vi "Get Waveform Name and Units.vi"(8 "Error In":errorcluster, 10 "CD Settings":T2={"CD Task Dependency"=18446744073709551615, "CD Task Dependency Ref"=18446744073709551615, "CD Task Available Wfms"=[], "CD Task Selected Wfms"=[], "Buffer Length (samples)"=0, "Min Enabled"=FALSE, "Max Enabled "=FALSE, "SP Enabled"=FALSE, "RMS Enabled"=FALSE, "Buffer Length (s)"=0.0, "Task Rate"=0.0, "Number of DAQ Chanels"=0} {"CD Task Dependency Ref" format="%.0x"; "CD Task Dependency" format="%.0x"}, 11 "CustomDevice Ref":T3 format="%.0x") -> (0 "Error Out":errorcluster, 4 "Waveform Channel Name and Units":T1(array[cluster]))   [LabVIEW 2017, in "Waveform-Processing-Custom-Device System Explorer.lvlib"]
doc: "This application will retrieve the channel names and units that were entered during the setup and configuration of the waveform input channels."
uses:
  Waveform-Processing-Custom-Device System Explorer.lvlib
  <vilib>/NI Veristand/Custom Device API/Custom Device Item Ref.ctl
  Shared/Custom Device Settings.ctl
  NationalInstruments.VeriStand.SystemStorage
  <vilib>/NI Veristand/Custom Device API/Custom Device API.lvlib
  <vilib>/NI VeriStand/Custom Device Tools/Custom Device Utility Library/Custom Device Utility Library.lvlib
  Shared/Waveform-Processing-Custom-Device Shared.lvlib
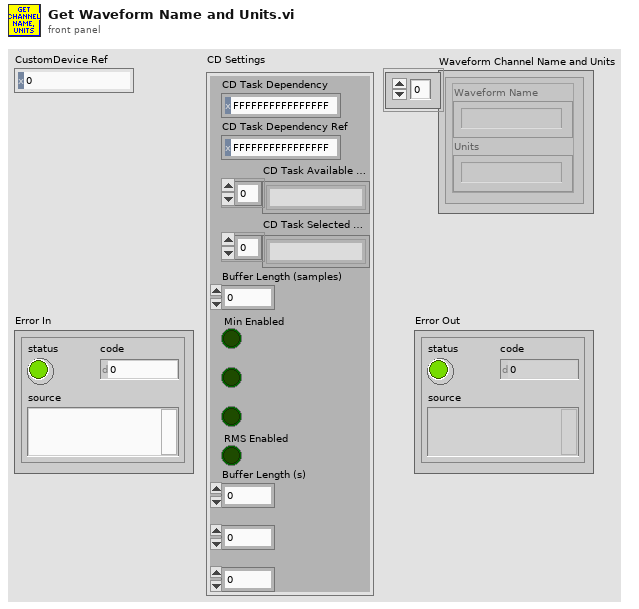
[diagram p1: front panel]
types:
  T1 = cluster{"Waveform Name":string, "Units":string}[]
  T2 = typedef "Waveform-Processing-Custom-Device Shared.lvlib/Custom Device Settings.ctl" = cluster{"CD Task Dependency":T3, "CD Task Dependency Ref":T3, "CD Task Available Wfms":string[], "CD Task Selected Wfms":string[], "Buffer Length (samples)":u32, "Min Enabled":bool, "Max Enabled ":bool, "SP Enabled":bool, "RMS Enabled":bool, "Buffer Length (s)":dbl, "Task Rate":dbl, "Number of DAQ Chanels":u32}
  T3 = typedef "Custom Device API.lvlib/Custom Device Item Ref.ctl" = u64
  T4 = typedef "Custom Device API.lvlib/Custom Device Pointer.ctl" = refnum<k24>
  T5 = typedef "Custom Device API.lvlib/Custom Device Waveform.ctl" = cluster{"Data Type":T6, "Units":string}
  T6 = typedef "Custom Device API.lvlib/Custom Device Waveform DataType.ctl" = enum16{"Double", "Complex Double"}
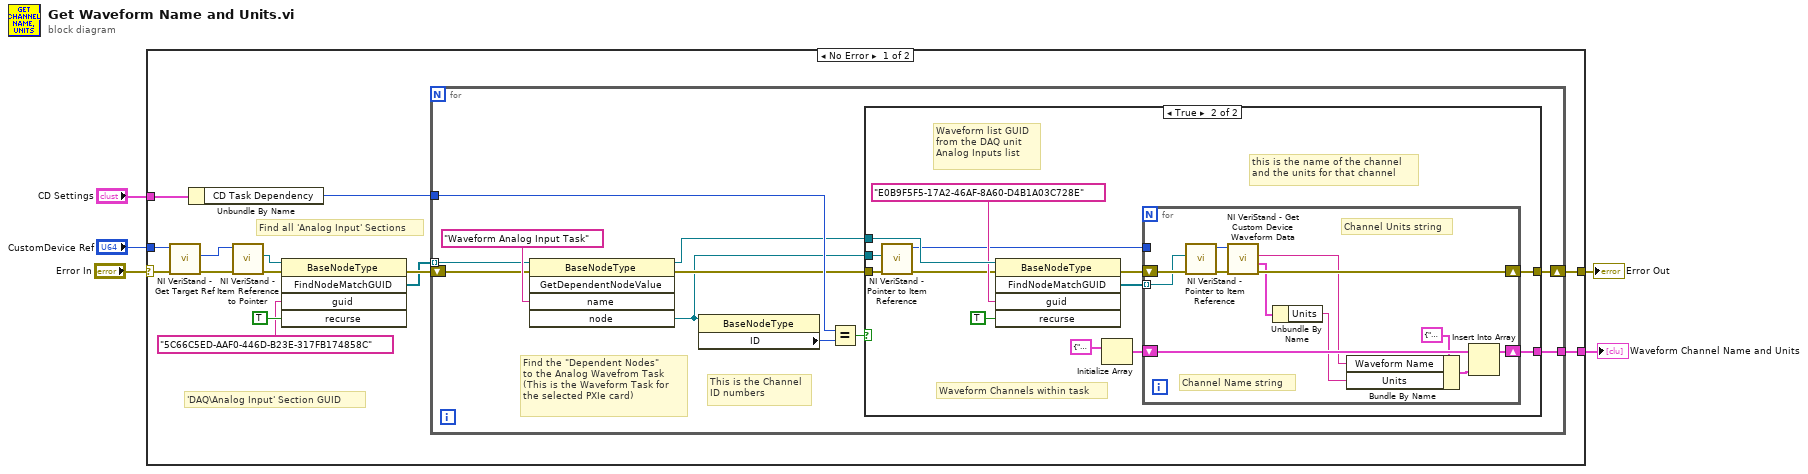
[diagram p0: block diagram]
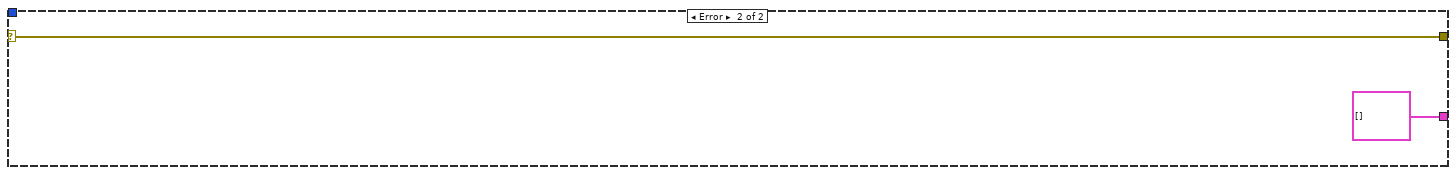
[diagram p3: hidden frame]
diagram:
  n1 = case shown="No Error" "Error In" {
    selector: "Error In" -> [w7 w58]
    tunnel: "CustomDevice Ref" -> [w13 _]
    tunnel: "CD Settings" -> [w10 _]
    tunnel: [w8 w58] -> w3
    tunnel: [w6 T1 []] -> w1
    frame No Error {
      # "'DAQ\\Analog Input' Section GUID"
      # "Find all 'Analog Input' Sections"
      n2 = call <vilib>:"NI VeriStand - Get Target Ref.vi"("error in"=w7, "Item Ref in"=w13) -> ("error out"=w14:errorcluster, "Target Ref"=w15:T3)  [unwired: 6 in, 2 out]
      n3 = Unbundle By Name(w10) -> ("CD Task Dependency"=w9:T3)
      n4 = call <vilib>:"NI VeriStand - Item Reference to Pointer.vi"("error in (no error)"=w14, "Item Ref in"=w15) -> ("error out"=w17:errorcluster, "Node Pointer"=w16:T4)  [unwired: 6 in, 2 out]
      n5 = invoke class="BaseNodeType" method="FindNodeMatchGUID"(reference=w16, error in=w17, "guid"="5C66C5ED-AAF0-446D-B23E-317FB174858C" ("Item GUID"), "recurse"=TRUE ("Find All? (T)")) -> (error out=w12:errorcluster, "FindNodeMatchGUID"=w11:refnum<k24>[])  [unwired: 1 in, 3 out]
      n6 = for {
        shift-right: [w22] -> w8
        shift-left: w12 -> [w28]
        tunnel: w11 -> [w27] mode=indexing
        tunnel: w9 -> [w26]
        tunnel: [w20] -> w6
        # "This is the Channel\nID numbers"
        # "Find the \"Dependent Nodes\" \nto the Analog Wavefrom Task\n(This is the Waveform Task for \nthe selected PXIe card)"
        n7 = invoke class="BaseNodeType" method="GetDependentNodeValue"(reference=w27, error in=w28, "name"="Waveform Analog Input Task" ("Property Name")) -> (reference out=w23:refnum<k24>, error out=w24:errorcluster, "node"=w21:refnum<k24>)  [unwired: 2 in, 2 out]
        n8 = property class="BaseNodeType"(reference=w21) -> ("ID"=w30:u64)  [unwired: 1 in, 2 out]
        n9 = Equal?(x=w26, y=w30) -> (x = y?=w25:bool)
        n10 = case shown="True" w25 {
          tunnel: w24 -> [w31 w41]
          tunnel: w23 -> [_ w43]
          tunnel: [w31 w37] -> w22
          tunnel: w21 -> [_ w39]
          tunnel: [_ w33] -> w20
          frame False {
          }
          frame True {
            # "this is the name of the channel \nand the units for that channel"
            # "Waveform list GUID\nfrom the DAQ unit\nAnalog Inputs list"
            # "Waveform Channels within task"
            n11 = call <vilib>:"NI VeriStand - Pointer to Item Reference.vi"("error in (no error)"=w41, "Node Pointer"=w39) -> ("error out"=w40:errorcluster, "Item Ref out"=w35:T3)  [unwired: 8 in]
            n12 = invoke class="BaseNodeType" method="FindNodeMatchGUID"(reference=w43, error in=w40, "guid"="E0B9F5F5-17A2-46AF-8A60-D4B1A03C728E", "recurse"=TRUE ("Find All? (T)")) -> (error out=w38:errorcluster, "FindNodeMatchGUID"=w36:refnum<k24>[])  [unwired: 1 in, 3 out]
            n13 = Initialize Array(cluster{"Waveform Name":string, "Units":string} {"Waveform Name"="", "Units"=""}) -> (w34:T1)  [unwired: 1 in]
            n14 = for {
              shift-right: [w48] -> w37
              shift-left: w38 -> [w52]
              tunnel: w36 -> [w51] mode=indexing
              tunnel: w35 -> [_]
              shift-right: [w55] -> w33
              shift-left: w34 -> [w56]
              # "Channel Units string"
              # "Channel Name string"
              n15 = call <vilib>:"NI VeriStand - Pointer to Item Reference.vi"("error in (no error)"=w52, "Node Pointer"=w51) -> ("error out"=w49:errorcluster, "Item Ref out"=w50:T3)  [unwired: 8 in]
              n16 = call <vilib>:"NI VeriStand - Get Custom Device Waveform Data.vi"("error in (no error)"=w49, "Waveform Ref in"=w50) -> ("error out"=w48:errorcluster, "Waveform"=w46:T5, "Waveform Name"=w47:string)  [unwired: 4 in, 3 out]
              n17 = Unbundle By Name(w46) -> ("Units"=w45:string)
              n18 = Bundle By Name(cluster=cluster{"Waveform Name":string, "Units":string} {"Waveform Name"="", "Units"=""}, "Waveform Name"=w47, "Units"=w45) -> (w53:cluster{"Waveform Name":string, "Units":string})
              n19 = Insert Into Array(array=w56, new element=w53) -> (w55:T1)  [unwired: 1 in]
            }
          }
        }
      }
    }
    frame Error {
    }
  }
  "Error Out" <- w3
  "Waveform Channel Name and Units" <- w1
